vi "_Load Config File.vi"(4 "error in (no error)":errorcluster) -> (0 "error out":errorcluster, 3 "Instrument":string[](array[string]))   [LabVIEW 2015]
uses:
  Type/_RT Command.ctl
  Type/_RT Configuration 2.ctl
  Configuration/_Global Configuration.vi
  <vilib>/Utility/config.llb/Read Key (I32).vi
  <vilib>/Utility/config.llb/Read Key (Boolean).vi
  <vilib>/Utility/config.llb/Read Key (String).vi
  <vilib>/Utility/config.llb/Write Key (String).vi
  <vilib>/Utility/config.llb/NI_LVConfig.lvlib
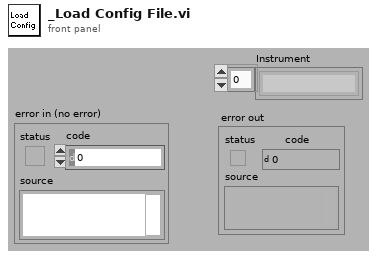
[diagram p1: front panel]
types:
  T1 = typedef "NI_LVConfig.lvlib/Config Data RefNum.ctl" = refnum<k1>
  T2 = typedef "_RT Command.ctl" = enum16{"Start", "Stop", "Runtime Update", "Get Data", "Get Info", "Get Status", "Get Param", "Get Config", "Get Table", "Read ADC", "Set Oscillator", "Update Config", "Update Table", "Set All Pol", "Set Pol and DC", "Set Max Mass", "Toggle RP", "Toggle EL", "Set PIC", "Initialize Turbo", "Send Turbo Comm", "Close Turbo", "P1", "P2", "P3", "Send Serial", "Set LC Out", "Get LC In", "Read VAC", "Test Table", "Toggle Power", "Get Startup", "Set Startup", "Get ADC Table", "Set ADC Table", "Get Brief Status", "Get Detail Status", "Auxiliary Update", "Set CC Logics", "Set CC Input Logics", "Ignore Error"}
  T3 = typedef "_RT Instrument 2.ctl" = cluster{"Table":T4[], "Instrument":string[]}
  T4 = typedef "_RT Configuration 2.ctl" = cluster{"Name":string, "Ch#":u8, "Min":dbl, "Max":dbl, "Def+":dbl, "Def-":dbl, "Offset":dbl, "Slope":dbl, "Type":u8, "Description":string, "SettleT":dbl}
  T5 = typedef "_Instrument Model.ctl" = enum16{"IONICS 3QA", "IONICS 3QB", "IONICS 3Q 110", "IONICS 3Q 120", "IONICS 3Q 210", "IONICS 3Q 220", "IONICS 3Q 310", "IONICS 3Q 320", "SHIMADZU LCMS-8080", "Simulation (Single Source)", "Simulation (Dual Source)"}
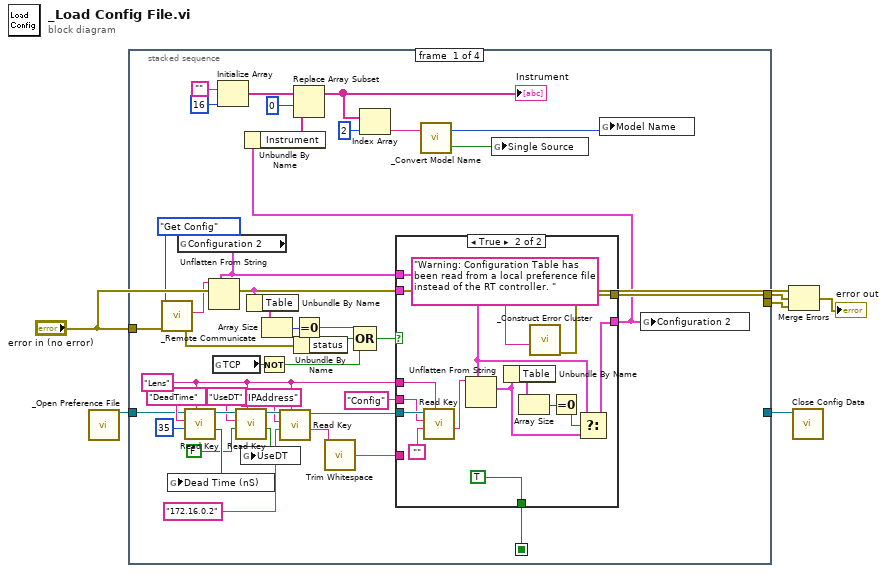
[diagram p0: block diagram]
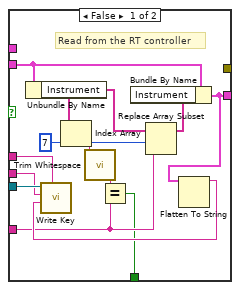
[diagram p2: hidden frame]
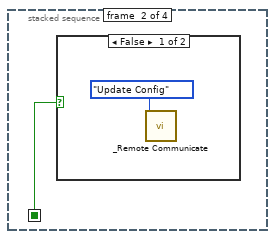
[diagram p3: hidden frame]
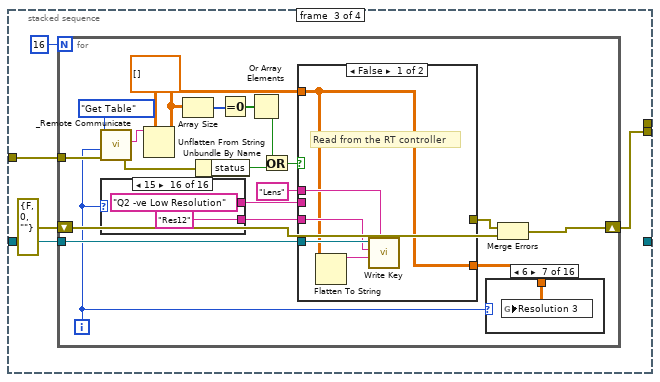
[diagram p5: hidden frame]
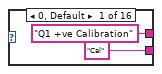
[diagram p6: hidden frame]
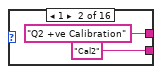
[diagram p7: hidden frame]
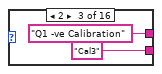
[diagram p8: hidden frame]
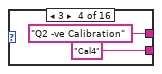
[diagram p9: hidden frame]
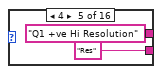
[diagram p10: hidden frame]
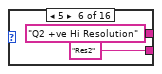
[diagram p11: hidden frame]
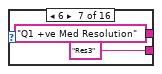
[diagram p12: hidden frame]
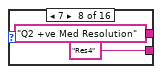
[diagram p13: hidden frame]
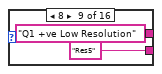
[diagram p14: hidden frame]
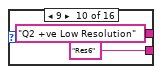
[diagram p15: hidden frame]
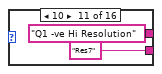
[diagram p16: hidden frame]
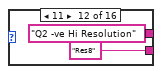
[diagram p17: hidden frame]
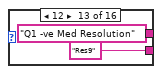
[diagram p18: hidden frame]
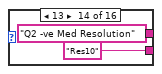
[diagram p19: hidden frame]
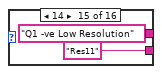
[diagram p20: hidden frame]
diagram:
  n1 = call "_Open Preference File.vi"() -> ("refnum"=w5:T1)  [unwired: 1 in, 6 out]
  n2 = stacked-sequence {
    seq-local: [w10 _ _ _] -> [_ w76 _ _]
    tunnel: [_ _ w79 _] -> w2
    tunnel: [w43 _ _ _] -> w3
    tunnel: w5 -> [w20 _ w82 w168]
    tunnel: [_ _ _ w167] -> w4
    tunnel: "error in (no error)" -> [w40 _ w80 w172]
    frame #0 {
      w15 = "Lens" ("section")
      n3 = call "_Remote Communicate.vi"("error in (no error)"=w40, "Command"=_RT_Command."Get Config") -> ("error out"=w47:errorcluster, "Info"=w42:string)  [unwired: 4 in, 2 out]
      n4 = global read "_Global Configuration.vi" "Configuration 2"() -> (w25:T3)
      n5 = call-poly <vilib>:"Read Key.vi"("section"=w15, "default value"=35, "key"="DeadTime", "refnum"=w20) -> ("value"=w39:i32, "refnum out"=w38:T1)  [unwired: 1 in, 5 out]
      n6 = global write "_Global Configuration.vi" "Dead Time (nS)"(w39) -> ()
      n7 = Unflatten From String(type=w25, binary string=w42) -> (value=w22:T3)  [unwired: 1 in, 4 out]
      n8 = global read "_Global Configuration.vi" "TCP"() -> (w19:bool)
      n9 = Initialize Array("", 16 ("dimension size")) -> (w29:string[])
      n10 = call-poly <vilib>:"Read Key.vi"("section"=w15, "default value"=FALSE, "key"="UseDT", "refnum"=w38) -> ("value"=w34:bool, "refnum out"=w17:T1)  [unwired: 1 in, 5 out]
      n11 = global write "_Global Configuration.vi" "UseDT"(w34) -> ()
      n12 = Unbundle By Name(w22) -> ("Table"=w24:T4[])
      n13 = Not(x=w19) -> (.not. x?=w18:bool)
      n14 = Array Size(array=w24) -> (size(s)=w23:i32)
      n15 = call-poly <vilib>:"Read Key.vi"("section"=w15, "default value"="172.16.0.2", "key"="IPAddress" ("section"), "refnum"=w17) -> ("value"=w12:string, "refnum out"=w16:T1)  [unwired: 2 in, 4 out]
      n16 = Equal To 0?(x=w23) -> (x = 0?=w21:bool)
      n17 = Unbundle By Name(w47) -> ("status"=w46:bool)
      n18 = call <vilib>:"Trim Whitespace.vi"("string"=w12) -> ("trimmed string"=w11:string)  [unwired: 1 in]
      n19 = Compound Arithmetic op=OR(w21, w46, w18) -> (w45:bool)
      n20 = case shown="True" w45 {
        tunnel: w22 -> [w58 _]
        tunnel: [w49 w63] -> w32
        tunnel: w16 -> [w61 w75]
        tunnel: w15 -> [w60 w72]
        tunnel: "Config" ("section") -> [w59 w70]
        tunnel: [_ w71] -> w43
        tunnel: w25 -> [_ w64]
        tunnel: w11 -> [w51 _]
        tunnel: [w50 TRUE] -> w10
        frame False {
          w54 = 7 ("index")
          # "Read from the RT controller"
          n21 = Unbundle By Name(w58) -> ("Instrument"=w55:string[])
          n22 = Index Array(array=w55, index=w54) -> (element=w53:string)
          n23 = call <vilib>:"Trim Whitespace.vi"("string"=w53) -> ("trimmed string"=w52:string)  [unwired: 1 in]
          n24 = Equal?(x=w52, y=w51) -> (x = y?=w50:bool)
          n25 = Replace Array Subset(array=w55, new element=w51, index=w54) -> (w57:string[])
          n26 = Bundle By Name(cluster=w58, "Instrument"=w57) -> (w49:T3)
          n27 = Flatten To String(anything=w49) -> (data string=w56:string)  [unwired: 1 in, 4 out]
          n28 = call-poly <vilib>:"Write Key.vi"("section"=w60, "value"=w56, "key"=w59, "refnum"=w61) -> ()  [unwired: 2 in, 6 out]
        }
        frame True {
          n29 = call-poly <vilib>:"Read Key.vi"("section"=w72, "default value"="", "key"=w70, "refnum"=w75) -> ("value"=w73:string)  [unwired: 2 in, 5 out]
          n30 = Unflatten From String(type=w64, binary string=w73) -> (value=w65:T3)  [unwired: 1 in, 4 out]
          n31 = Unbundle By Name(w65) -> ("Table"=w67:T4[])
          n32 = Array Size(array=w67) -> (size(s)=w68:i32)
          n33 = call "_Construct Error Cluster.vi"("reason"="Warning: Configuration Table has been read from a local preference file instead of the RT controller. ") -> ("error out"=w71:errorcluster)  [unwired: 3 in, 3 out]
          n34 = Equal To 0?(x=w68) -> (x = 0?=w66:bool)
          n35 = Select(t=w64, s=w66, f=w65) -> (s? t:f=w63:T3)
        }
      }
      n36 = Unbundle By Name(w32) -> ("Instrument"=w27:string[])
      n37 = Replace Array Subset(array=w29, new element=w27, index=0) -> (w26:string[])
      "Instrument" <- w26
      n38 = Index Array(array=w26, index=2) -> (element=w9:string)
      n39 = call "_Convert Model Name.vi"("Model"=w9) -> ("SingleSource"=w8:bool, "Model Name"=w7:T5)  [unwired: 1 in]
      n40 = global write "_Global Configuration.vi" "Single Source"(w8) -> ()
      n41 = global write "_Global Configuration.vi" "Model Name"(w7) -> ()
      n42 = global write "_Global Configuration.vi" "Configuration 2"(w32) -> ()
    }
    frame #1 {
      n43 = case shown="False" w76 {
        frame False {
          n44 = call "_Remote Communicate.vi"("Command"=_RT_Command."Update Config") -> ()  [unwired: 5 in, 4 out]
        }
        frame True {
        }
      }
    }
    frame #2 {
      n45 = for {
        N: 16 -> [_]
        tunnel: w82 -> [w101]
        tunnel: w80 -> [w100]
        shift-right: [w87] -> w79
        shift-left: errorcluster {"status"=FALSE, "code"=0, "source"=""} ("error out") -> [w88]
        i -> [w85]
        n46 = call "_Remote Communicate.vi"("error in (no error)"=w100, "DC Param"=w85, "Command"=_RT_Command."Get Table") -> ("error out"=w90:errorcluster, "Info"=w99:string)  [unwired: 3 in, 2 out]
        n47 = case shown="15" w85 {
          tunnel: ["Q1 +ve Calibration" ("section") "Q2 +ve Calibration" ("section") "Q1 -ve Calibration" ("section") "Q2 -ve Calibration" ("section") "Q1 +ve Hi Resolution" ("section") "Q2 +ve Hi Resolution" ("section") "Q1 +ve Med Resolution" ("section") "Q2 +ve Med Resolution" ("section") "Q1 +ve Low Resolution" ("section") "Q2 +ve Low Resolution" ("section") "Q1 -ve Hi Resolution" ("section") "Q2 -ve Hi Resolution" ("section") "Q1 -ve Med Resolution" ("section") "Q2 -ve Med Resolution" ("section") "Q1 -ve Low Resolution" ("section") "Q2 -ve Low Resolution" ("section")] -> w83
          tunnel: ["Cal" ("section") "Cal2" ("section") "Cal3" ("section") "Cal4" ("section") "Res" ("section") "Res2" ("section") "Res3" ("section") "Res4" ("section") "Res5" ("section") "Res6" ("section") "Res7" ("section") "Res8" ("section") "Res9" ("section") "Res10" ("section") "Res11" ("section") "Res12" ("section")] -> w84
          frame 0, Default {
          }
          frame 1 {
          }
          frame 2 {
          }
          frame 3 {
          }
          frame 4 {
          }
          frame 5 {
          }
          frame 6 {
          }
          frame 7 {
          }
          frame 8 {
          }
          frame 9 {
          }
          frame 10 {
          }
          frame 11 {
          }
          frame 12 {
          }
          frame 13 {
          }
          frame 14 {
          }
          frame 15 {
          }
        }
        n48 = Unflatten From String(type=dbl[][] [] ("Cal-"), binary string=w99) -> (value=w91:dbl[][])  [unwired: 1 in, 4 out]
        n49 = Array Size(array=w91) -> (size(s)=w94:i32[])
        n50 = Unbundle By Name(w90) -> ("status"=w97:bool)
        n51 = Equal To 0?(x=w94) -> (x = 0?=w93:bool[])
        n52 = Or Array Elements(Boolean array=w93) -> (logical OR=w92:bool)
        n53 = Or(x=w92, y=w97) -> (x .or. y?=w96:bool)
        n54 = case shown="False" w96 {
          tunnel: [w152 w164] -> w86
          tunnel: w101 -> [w155 w166]
          tunnel: "Lens" ("section") -> [w154 w162]
          tunnel: w84 -> [w153 w160]
          tunnel: [_ w161] -> w89
          tunnel: w91 -> [w152 w159]
          tunnel: w83 -> [_ w158]
          frame False {
            # "Read from the RT controller"
            n55 = Flatten To String(anything=w152) -> (data string=w151:string)  [unwired: 1 in, 4 out]
            n56 = call-poly <vilib>:"Write Key.vi"("section"=w154, "value"=w151, "key"=w153, "refnum"=w155) -> ()  [unwired: 2 in, 6 out]
          }
          frame True {
            n57 = call-poly <vilib>:"Read Key.vi"("section"=w162, "default value"="", "key"=w160, "refnum"=w166) -> ("value"=w163:string)  [unwired: 2 in, 5 out]
            n58 = Format Into String(format string="Warning: %s Table has been read from a local preference file instead of the RT controller. ", w158) -> (resulting string=w156:string)  [unwired: 2 in, 1 out]
            n59 = Unflatten From String(type=w159, binary string=w163) -> (value=w164:dbl[][])  [unwired: 1 in, 4 out]
            n60 = call "_Construct Error Cluster.vi"("reason"=w156) -> ("error out"=w161:errorcluster)  [unwired: 3 in, 3 out]
          }
        }
        n61 = case shown="6" w85 {
          tunnel: w86 -> [w135 w136 w137 w138 w139 w140 w141 w142 w143 w144 w145 w146 w147 w148 w149 w150]
          frame 0, Default {
            n62 = global write "_Global Configuration.vi" "Calibration"(w135) -> ()
          }
          frame 1 {
            n63 = global write "_Global Configuration.vi" "Calibration 2"(w136) -> ()
          }
          frame 2 {
            n64 = global write "_Global Configuration.vi" "Calibration 3"(w137) -> ()
          }
          frame 3 {
            n65 = global write "_Global Configuration.vi" "Calibration 4"(w138) -> ()
          }
          frame 4 {
            n66 = global write "_Global Configuration.vi" "Resolution"(w139) -> ()
          }
          frame 5 {
            n67 = global write "_Global Configuration.vi" "Resolution 2"(w140) -> ()
          }
          frame 6 {
            n68 = global write "_Global Configuration.vi" "Resolution 3"(w141) -> ()
          }
          frame 7 {
            n69 = global write "_Global Configuration.vi" "Resolution 4"(w142) -> ()
          }
          frame 8 {
            n70 = global write "_Global Configuration.vi" "Resolution 5"(w143) -> ()
          }
          frame 9 {
            n71 = global write "_Global Configuration.vi" "Resolution 6"(w144) -> ()
          }
          frame 10 {
            n72 = global write "_Global Configuration.vi" "Resolution 7"(w145) -> ()
          }
          frame 11 {
            n73 = global write "_Global Configuration.vi" "Resolution 8"(w146) -> ()
          }
          frame 12 {
            n74 = global write "_Global Configuration.vi" "Resolution 9"(w147) -> ()
          }
          frame 13 {
            n75 = global write "_Global Configuration.vi" "Resolution 10"(w148) -> ()
          }
          frame 14 {
            n76 = global write "_Global Configuration.vi" "Resolution 11"(w149) -> ()
          }
          frame 15 {
            n77 = global write "_Global Configuration.vi" "Resolution 12"(w150) -> ()
          }
        }
        n78 = Merge Errors(w89, w88) -> (w87:errorcluster)
      }
    }
    frame #3 {
      w173 = T4[] []  # ADC Table
      n79 = call "_Remote Communicate.vi"("error in (no error)"=w172, "Command"=_RT_Command."Get ADC Table") -> ("Info"=w174:string)  [unwired: 4 in, 3 out]
      n80 = Unflatten From String(type=w173, binary string=w174) -> (value=w169:T4[])  [unwired: 1 in, 4 out]
      n81 = Array Size(array=w169) -> (size(s)=w171:i32)
      n82 = Greater Than 0?(x=w171) -> (x > 0?=w170:bool)
      n83 = case shown="True" w170 {
        tunnel: w169 -> [_ w179]
        tunnel: w168 -> [w176 w178]
        tunnel: [w176 w177] -> w167
        frame False {
        }
        frame True {
          n84 = for {
            tunnel: w179 -> [w196] mode=indexing
            tunnel: w178 -> [w183]
            tunnel: [w180] -> w177
            i -> [w182]
            w186 = "0"
            w191 = i16 3 ("precision (6)")
            n85 = Unbundle By Name(w196) -> ("Name"=w189:string, "Offset"=w195:dbl, "Slope"=w194:dbl, "Min"=w193:dbl, "Max"=w192:dbl)
            n86 = Number To Decimal String(number=w182) -> (decimal integer string=w190:string)  [unwired: 1 out]
            n87 = Number To Fractional String(number=w195) -> (F-format string=w188:string)  [unwired: 3 out]
            n88 = Number To Fractional String(number=w194) -> (F-format string=w187:string)  [unwired: 3 out]
            n89 = Number To Fractional String(number=w193, precision (6)=w191) -> (F-format string=w185:string)  [unwired: 2 out]
            n90 = Number To Fractional String(number=w192, precision (6)=w191) -> (F-format string=w184:string)  [unwired: 2 out]
            n91 = Build Array(w190, w189, w186, w188, w187, w186, w185, w184) -> (w181:string[])
            n92 = for {
              tunnel: w183 -> [w204]
              tunnel: w182 -> [w202]
              tunnel: w181 -> [w198] mode=indexing
              tunnel: [w197] -> w180
              i -> [w203]
              n93 = Format Into String(format string="Row%d-Col%d" ("section"), w202, w203) -> (resulting string=w200:string)  [unwired: 2 in, 1 out]
              n94 = call-poly <vilib>:"Write Key.vi"("section"="ADC", "value"=w198, "key"=w200, "refnum"=w204) -> ("refnum out"=w197:T1)  [unwired: 2 in, 5 out]
            }
          }
        }
      }
    }
  }
  n95 = Merge Errors("error in (no error)", w3, w2) -> (→"error out":errorcluster)
  n96 = call <vilib>:"Close Config Data.vi"("refnum"=w4) -> ()  [unwired: 2 in, 9 out]
